vi "HEWH Errors Save to File.vi"(0 "EEV Over A":bool, 1 "T-OUT Over A":bool, 2 "TR number":string) -> (7 "Output File Name":string)   [LabVIEW 2016]
doc: "This VI logs errors (EEV limit and T-OUT limit) to file. Each error is saved to file (Errors.csv) that includes information about the date recorded, error type, and TR #."
uses:
  <vilib>/Utility/file.llb/Write To Spreadsheet File (DBL).vi
  <vilib>/Utility/file.llb/Write To Spreadsheet File (string).vi
panel:
  out "new file path":path
  out "output array":string[][](array[string])
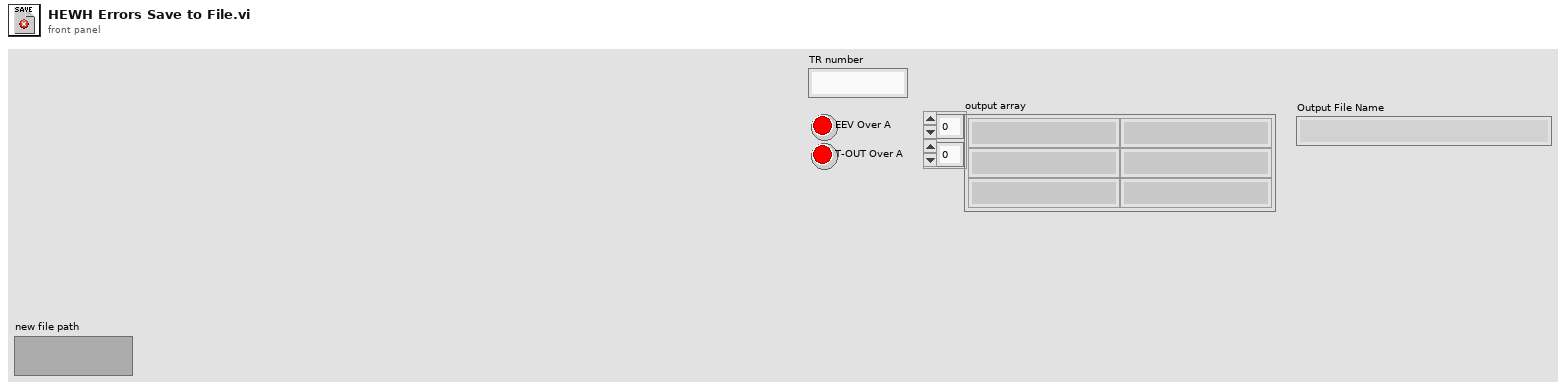
[diagram p1: front panel]
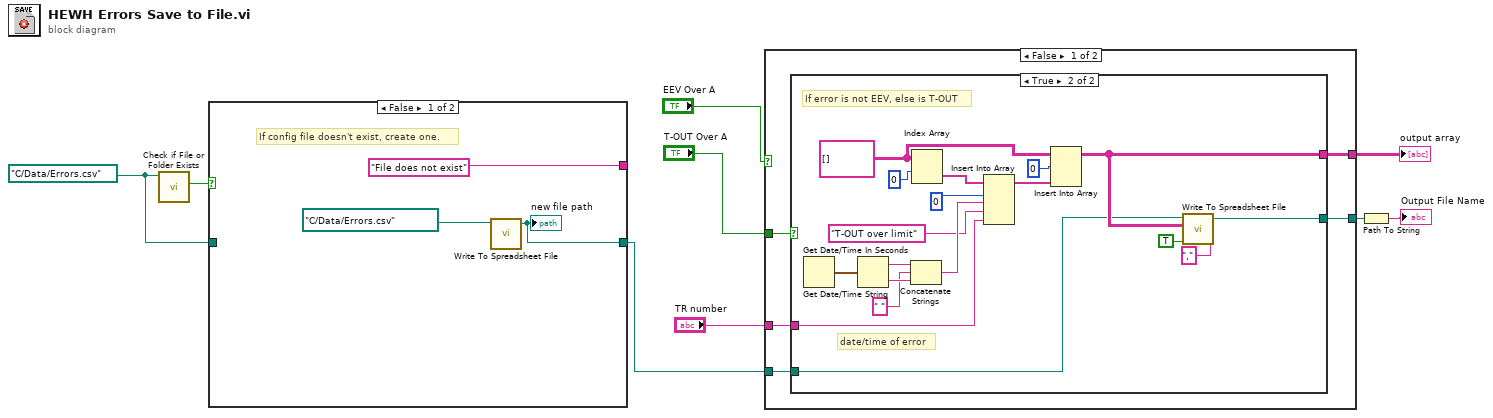
[diagram p0: block diagram]
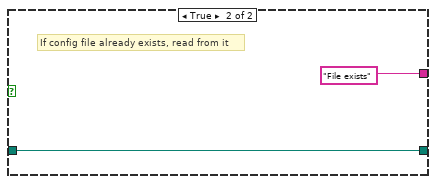
[diagram p2: hidden frame]
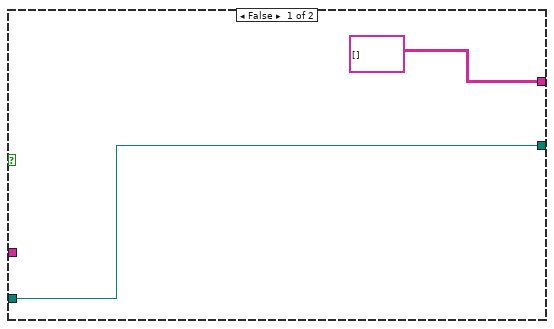
[diagram p3: hidden frame]
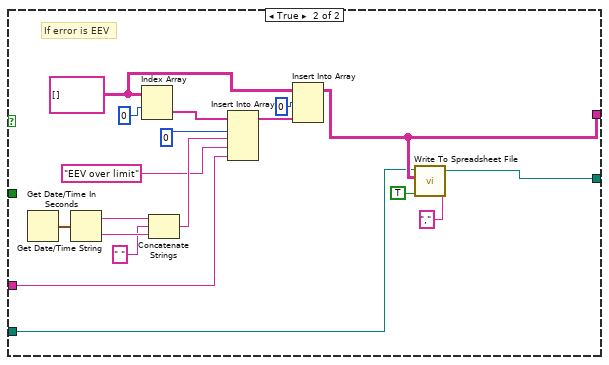
[diagram p4: hidden frame]
diagram:
  w2 = path "C:/Data/Errors.csv" ("file path (use dialog)")
  n1 = call <vilib>:"Check if File or Folder Exists.vi"("path"=w2) -> ("file or folder exists?"=w3:bool)  [unwired: 8 in, 2 out]
  n2 = case shown="False" w3 {
    tunnel: ["File does not exist" "File exists"] -> _
    tunnel: w2 -> [_ w13]
    tunnel: [w10 w13] -> w1
    frame False {
      # "If config file doesn't exist, create one."
      n3 = call-poly <vilib>:"Write To Spreadsheet File.vi"("file path (dialog if empty)"=path "C:/Data/Errors.csv" ("file path (use dialog)")) -> ("new file path (Not A Path if cancelled)"=w10:path)  [unwired: 7 in]
      "new file path" <- w10
    }
    frame True {
      # "If config file already exists, read from it"
    }
  }
  n4 = case shown="False" "EEV Over A" {
    tunnel: "T-OUT Over A" -> [w19 _]
    tunnel: [w18 w45] -> w9
    tunnel: [w17 w44] -> w8
    tunnel: "TR number" -> [w16 w42]
    tunnel: w1 -> [w15 w43]
    frame False {
      n5 = case shown="True" w19 {
        tunnel: [string[][] [] w27] -> w18
        tunnel: [w20 w26] -> w17
        tunnel: w16 -> [_ w25]
        tunnel: w15 -> [w20 w24]
        frame False {
        }
        frame True {
          w32 = string[][] []
          # "date/time of error"
          # "If error is not EEV, else is T-OUT"
          n6 = Get Date/Time In Seconds() -> (seconds since 1Jan1904=w38:timestamp)
          n7 = Get Date/Time String(seconds (now)=w38) -> (date string=w39:string, time string=w30:string)  [unwired: 2 in]
          n8 = Concatenate Strings(w39, " " ("string"), w30) -> (w34:string)
          n9 = Index Array(array=w32, index (row)=0 ("disabled index (col)")) -> (element=w36:string[])  [unwired: 1 in]
          n10 = Insert Into Array(array=w36, index=0, new element #1=w34, new element #2="T-OUT over limit", new element #3=w25) -> (w33:string[])
          n11 = Insert Into Array(array=w32, index (row)=0, new element=w33) -> (w27:string[][])  [unwired: 1 in]
          n12 = call-poly <vilib>:"Write To Spreadsheet File.vi"("delimiter (\\t)"="," ("delimiter (\\t)"), "append to file? (new file:F)"=TRUE, "2D data"=w27, "file path (dialog if empty)"=w24) -> ("new file path (Not A Path if cancelled)"=w26:path)  [unwired: 4 in]
        }
      }
    }
    frame True {
      w49 = string[][] []
      # "If error is EEV"
      n13 = Get Date/Time In Seconds() -> (seconds since 1Jan1904=w56:timestamp)
      n14 = Get Date/Time String(seconds (now)=w56) -> (date string=w57:string, time string=w47:string)  [unwired: 2 in]
      n15 = Index Array(array=w49, index (row)=0 ("disabled index (col)")) -> (element=w54:string[])  [unwired: 1 in]
      n16 = Concatenate Strings(w57, " " ("string"), w47) -> (w52:string)
      n17 = Insert Into Array(array=w54, index=0, new element #1=w52, new element #2="EEV over limit", new element #3=w42) -> (w50:string[])
      n18 = Insert Into Array(array=w49, index (row)=0, new element=w50) -> (w45:string[][])  [unwired: 1 in]
      n19 = call-poly <vilib>:"Write To Spreadsheet File.vi"("delimiter (\\t)"="," ("delimiter (\\t)"), "append to file? (new file:F)"=TRUE, "2D data"=w45, "file path (dialog if empty)"=w43) -> ("new file path (Not A Path if cancelled)"=w44:path)  [unwired: 4 in]
    }
  }
  "output array" <- w9
  n20 = Path To String(path=w8) -> (string=→"Output File Name":string)
